vi "Query.vi"(8 "error in (no error)":errorcluster, 9 "current time":timestamp, 10 "gRPCid":T1) -> (0 "error out":errorcluster)   [LabVIEW 2019, in "ctet_dio_User Library.lvlib"]
uses:
  ctet_dio_User Library.lvlib
  Servers/ctet_dio/gRPC lvSupport/Server API/typeDefs/grpcId.ctl
  Servers/ctet_dio/ctet_dio Class/RPC Messages/measurementservice_QueryResponse/measurementservice_QueryResponse_Data.ctl
  Servers/ctet_dio/ctet_dio Class/ctet_dio.lvclass
  Servers/ctet_dio/gRPC lvSupport/gprc-lvsupport.lvlib
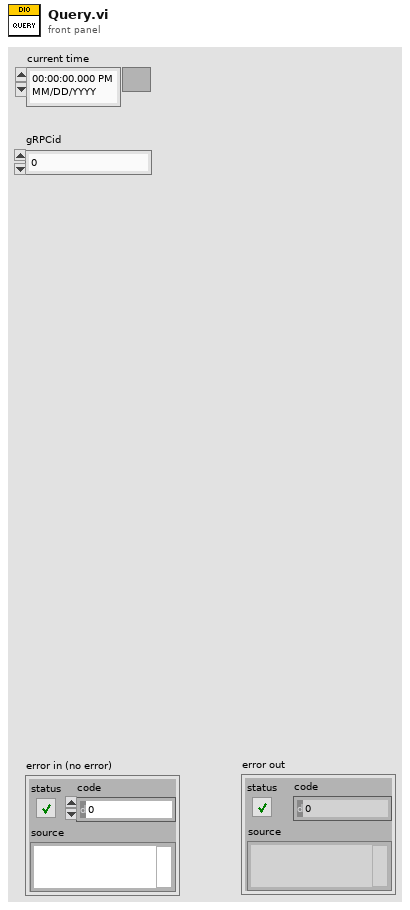
[diagram p1: front panel]
types:
  T1 = typedef "ctet_dio.lvlib/gprc-lvsupport.lvlib/grpcId.ctl" = u64
  T2 = typedef "ctet_dio.lvlib/ctet_dio.lvclass/measurementservice_QueryResponse_Data.ctl" = cluster{"message":string, "status":i64}
  T3 = typedef "ctet_dio.lvlib/ctet_dio.lvclass/measurementservice_QueryRequest_Data.ctl" = cluster{"query":string}
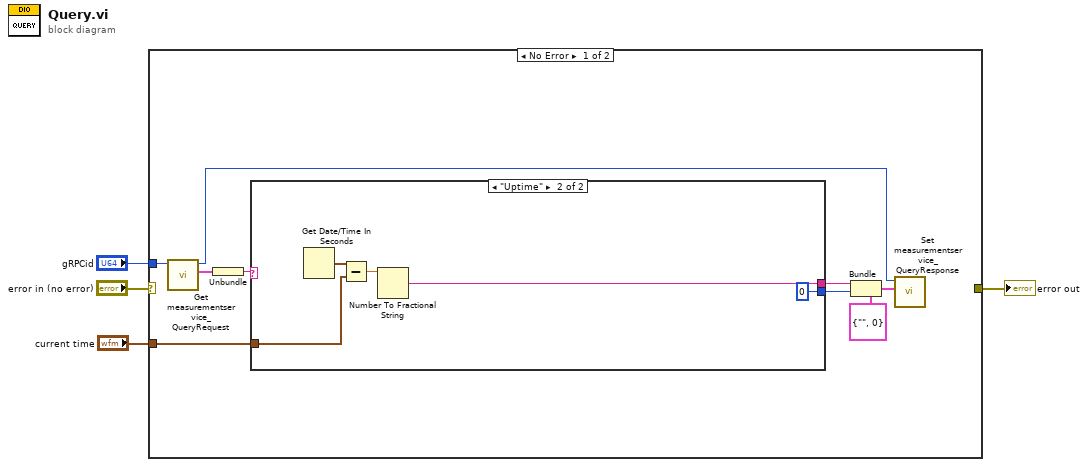
[diagram p0: block diagram]
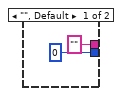
[diagram p2: hidden frame]
diagram:
  n1 = case shown="No Error" "error in (no error)" {
    selector: "error in (no error)" -> [_ w21]
    tunnel: [_ w21] -> w4
    tunnel: "current time" -> [w13 _]
    tunnel: "gRPCid" -> [w10 _]
    frame No Error {
      n2 = call "Get measurementservice_QueryRequest.vi"("gRPCid"=w10) -> ("Message Data"=w9:T3, "gRPCid out"=w5:T1)  [unwired: 8 in, 1 out]
      n3 = Unbundle(w9) -> ("query"=w8:string)
      n4 = case shown="\"Uptime\"" w8 {
        tunnel: w13 -> [_ w19]
        tunnel: ["" w17] -> w12
        tunnel: [i64 0 ("status") i64 0 ("status")] -> w11
        frame "", Default {
        }
        frame "Uptime" {
          n5 = Get Date/Time In Seconds() -> (seconds since 1Jan1904=w20:timestamp)
          n6 = Subtract(x=w20, y=w19) -> (x-y=w18:dbl)
          n7 = Number To Fractional String(number=w18) -> (F-format string=w17:string)  [unwired: 3 in]
        }
      }
      n8 = Bundle(cluster=T2 {"message"="", "status"=0} ("measurementservice_QueryResponse_Data"), "message"=w12, "status"=w11) -> (w6:T2)
      n9 = call "Set measurementservice_QueryResponse.vi"("Message Data"=w6, "gRPCid"=w5) -> ()  [unwired: 9 in, 1 out]
    }
    frame Error {
    }
  }
  "error out" <- w4
